vi "Fatten5.vi"(10 "GIC Input":T1={"Real/Sim"=FALSE, "WP Lats and Longs"={"WP Lats"=[], "WP Longs"=[]}, "GPS Time Int"=0.0, "GPS Com Port"="", "Compass Com Port"="", "Prop Com Port"="", "GPS Data"=[], "Compass"=0.0, "LMS Vector"=[], "Vision Vector"=[], "Direction Cmd"=0.0, "Speed Cmd"=0.0, "Time of Last GPS"=0.0, "WP Vector"=[], "WP Number"=0, "Num of WPs"=0, "SW Map"=[], "Obst Lats and Longs"={"Obst Lats"=[], "Obst Longs"=[]}, "Parameters"=[], "Path Cluster"={"Path x nodes"=[], "Path y nodes"=[]}, "     Use ?\nOff       On"=[TRUE, TRUE, FALSE, FALSE]} {"Obst Lats and Longs"."Obst Longs" format="%#_8g"; "Obst Lats and Longs"."Obst Lats" format="%#_8g"}) -> (2 "GIC Output":T1={"Real/Sim"=FALSE, "WP Lats and Longs"={"WP Lats"=[], "WP Longs"=[]}, "GPS Time Int"=0.0, "GPS Com Port"="", "Compass Com Port"="", "Prop Com Port"="", "GPS Data"=[], "Compass"=0.0, "LMS Vector"=[], "Vision Vector"=[], "Direction Cmd"=0.0, "Speed Cmd"=0.0, "Time of Last GPS"=0.0, "WP Vector"=[], "WP Number"=0, "Num of WPs"=0, "SW Map"=[], "Obst Lats and Longs"={"Obst Lats"=[], "Obst Longs"=[]}, "Parameters"=[], "Path Cluster"={"Path x nodes"=[], "Path y nodes"=[]}, "     Use ?\nOff       On"=[TRUE, TRUE, FALSE, FALSE]} {"Obst Lats and Longs"."Obst Longs" format="%#_8g"; "Obst Lats and Longs"."Obst Lats" format="%#_8g"})   [LabVIEW 2014]
panel:
  out "Array":dbl[](array[numeric])
  out "Numeric":dbl
  out "Test SWMap Out":dbl[][](array[numeric])
  in  "Test Fat":dbl=1.0
  # "Fatten"
  # "GPS"
  # "LMS"
  # "Vision"
  # "Prop"
  # "GPS"
  # "LMS"
  # "Vision"
  # "Prop"
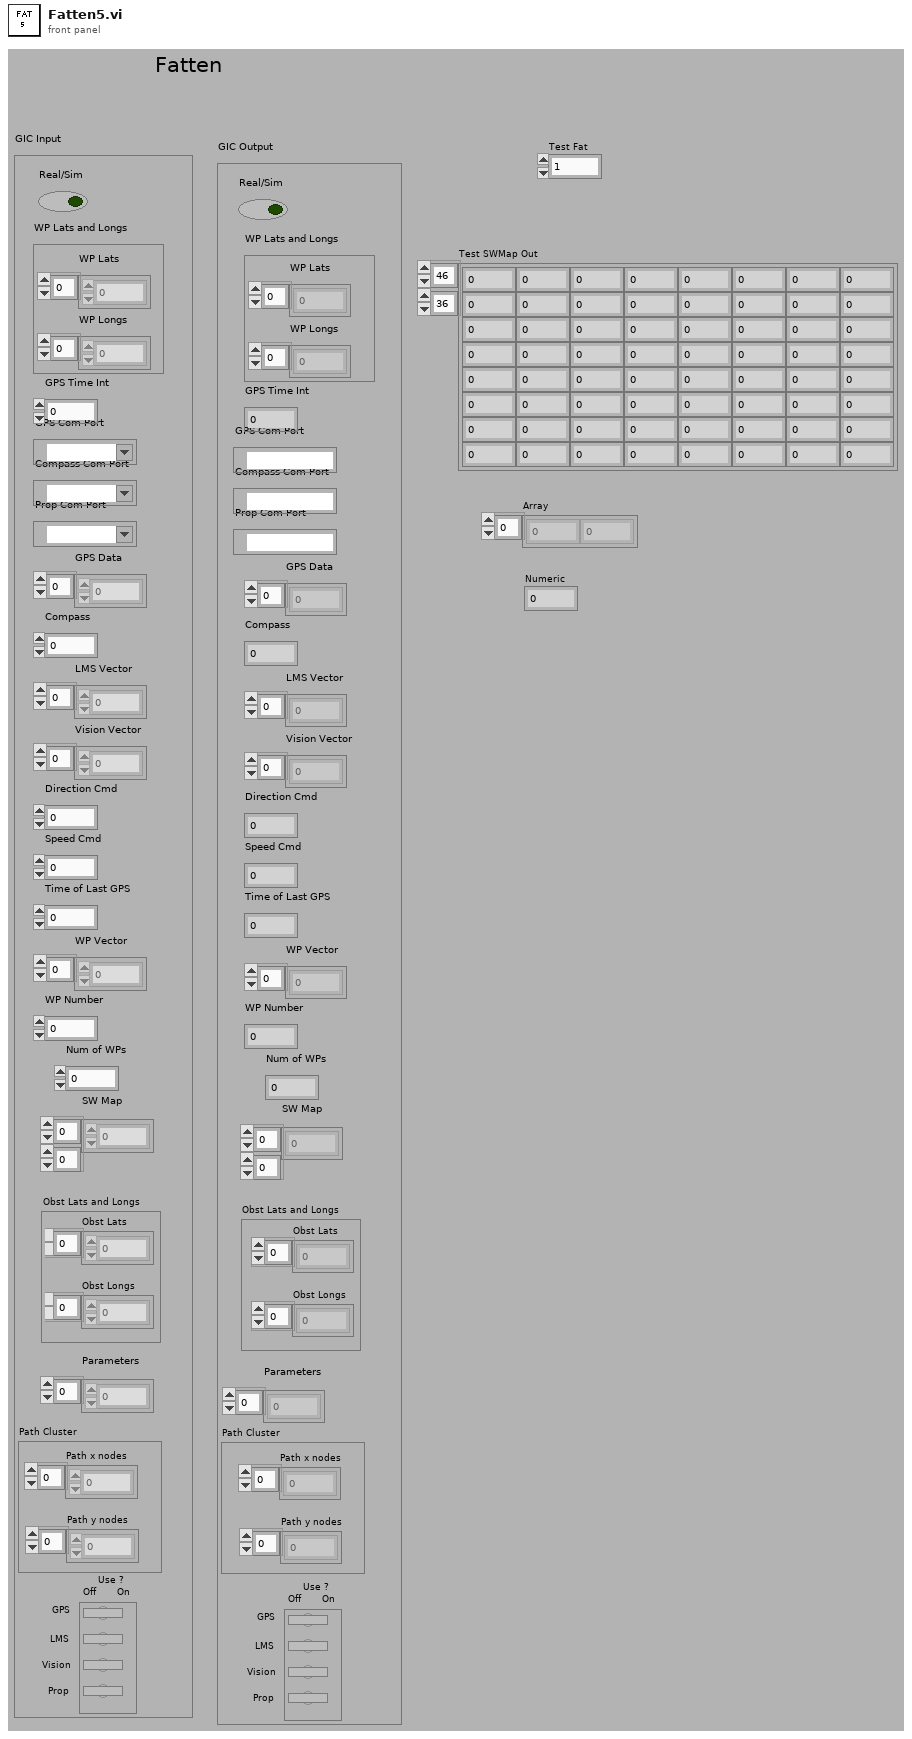
[diagram p1: front panel]
types:
  T1 = cluster{"Real/Sim":bool, "WP Lats and Longs":cluster{"WP Lats":dbl[], "WP Longs":dbl[]}, "GPS Time Int":dbl, "GPS Com Port":refnum<visa-resource-name>, "Compass Com Port":refnum<visa-resource-name>, "Prop Com Port":refnum<visa-resource-name>, "GPS Data":dbl[], "Compass":dbl, "LMS Vector":dbl[], "Vision Vector":dbl[], "Direction Cmd":dbl, "Speed Cmd":dbl, "Time of Last GPS":dbl, "WP Vector":dbl[], "WP Number":i32, "Num of WPs":i16, "SW Map":i32[][], "Obst Lats and Longs":cluster{"Obst Lats":dbl[], "Obst Longs":dbl[]}, "Parameters":dbl[], "Path Cluster":cluster{"Path x nodes":dbl[], "Path y nodes":dbl[]}, "     Use ?\nOff       On":bool[]}
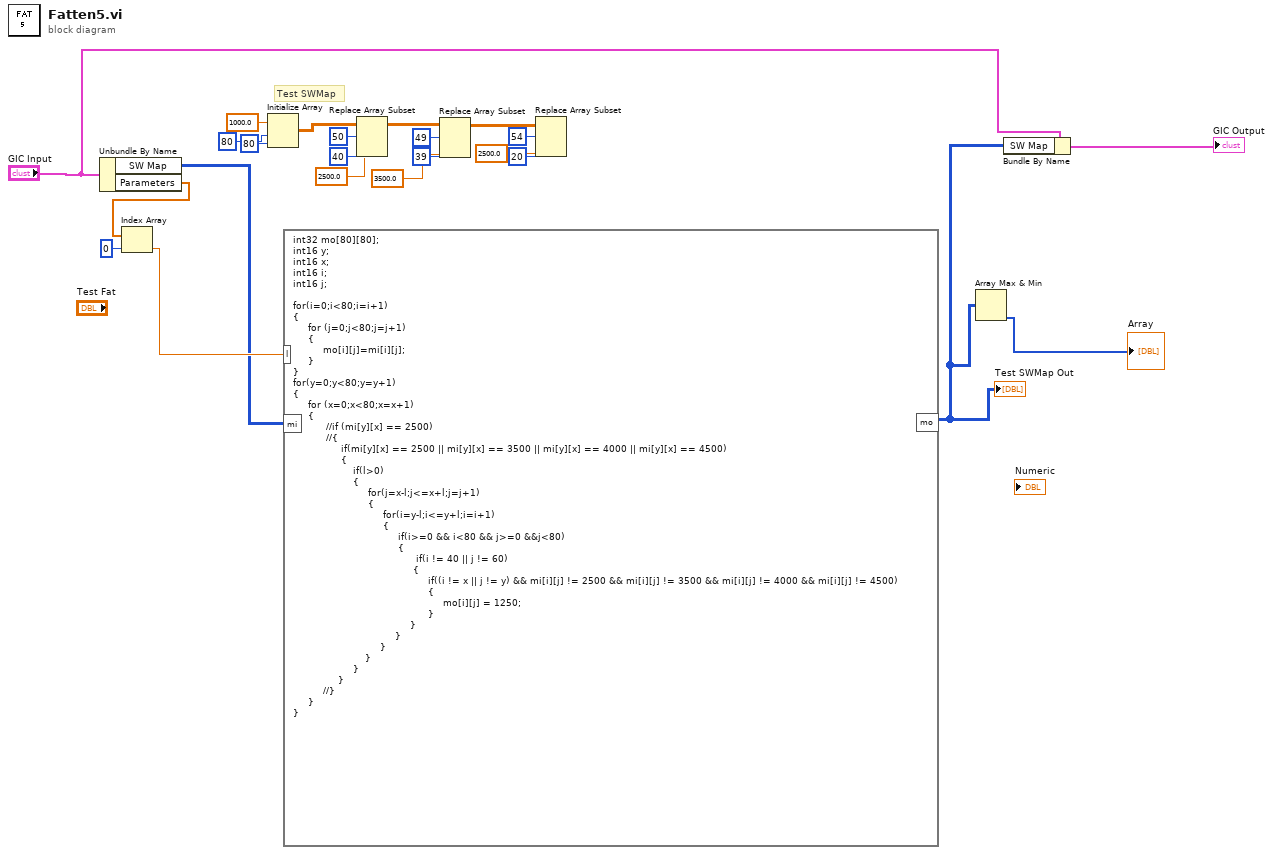
[diagram p0: block diagram]
diagram:
  # "Test SWMap"
  n1 = Unbundle By Name("GIC Input") -> ("SW Map"=w1:i32[][], "Parameters"=w12:dbl[])
  n2 = Index Array(array=w12, index=0) -> (element=w2:dbl)
  n3 = Initialize Array(1000.0 ("element"), 80 ("dimension size"), 80 ("dimension size")) -> (w20:dbl[][])
  n4 = formula code="int32 mo[80][80];\nint16 y;\nint16 x;\nint16 i;\nint16 j;\n\nfor(i=0;i<80;i=i+1)\n{\n     for (j=0;j<80;j=j+1)\n     {\n          mo[i][j]=mi[i][j];\n     }\n}\nfor(y=0;y<80;y=y+1)\n{\n     for (x=0;x<80;x=x+1)\n     {\n           //if (mi[y][x] == 2500)\n           //{\n                if(mi[y][x] == 2500 || mi[y][x] == 3500 || mi[y][x] == 4000 || mi[y][x] == 4500)\n                {\n                    if(l>0)\n                    {\n                         for(j=x-l;j<=x+l;j=j+1)\n                         {\n                              for(i=y-l;i<=y+l;i=i+1)\n                              {\n                                   if(i>=0 && i<80 && j>=0 &&j<80)\n                                   {\n                                         if(i != 40 || j != 60)\n                                        {\n                                             if((i != x || j != y) && mi[i][j] != 2500 && mi[i][j] != 3500 && mi[i][j] != 4000 && mi[i][j] != 4500)\n                                             {\n                                                  mo[i][j] = 1250;\n                                             }\n                                       }\n                                  }\n                             }\n                        }\n                    }\n               } \n          //}\n     }\n}"("mi"=w1, "l"=w2) -> ("mo"=w3:i32[][])
  "Test SWMap Out" <- w3
  n5 = Replace Array Subset(array=w20, new element=2500.0 ("new element/subarray"), index (row)=50, index (col)=40 ("disabled index (col)")) -> (w16:dbl[][])
  n6 = Replace Array Subset(array=w16, new element=3500.0 ("new element/subarray"), index (row)=49, index (col)=39 ("disabled index (col)")) -> (w9:dbl[][])
  n7 = Replace Array Subset(array=w9, new element=2500.0 ("new element/subarray"), index (row)=54, index (col)=20 ("disabled index (col)")) -> ()  [unwired: 1 out]
  n8 = Array Max & Min(array=w3) -> (min index (indices)=→"Array":i32[])  [unwired: 3 out]
  n9 = Bundle By Name(cluster="GIC Input", "SW Map"=w3) -> (→"GIC Output":T1)
